vi "SPI Set Frame Size.vi"(8 "Error In":errorcluster, 9 "Frame Size (Bytes)":u8, 10 "SPI Channel (0)":u8, 11 "LINX Device Config":T1) -> (0 "Error Out":errorcluster, 3 "LINX Device Config":T1)   [LabVIEW 2020, in "LMH-LINX.lvlib" / "Device.lvlib"]
doc: "Set the frame size in bytes for the specified SPI Channel."
uses:
  Device.lvlib
  Type Defs/LINX Device Config.ctl
  Type Defs/Interface.ctl
  Type Defs/TCP Config.ctl
  Type Defs/Channels.ctl
  Type Defs/Error Type.ctl
  LMH-LINX.lvlib
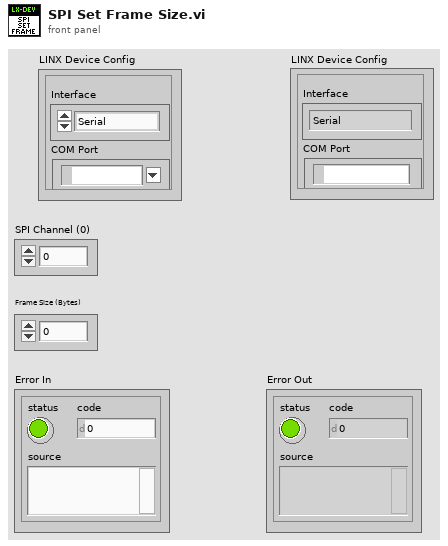
[diagram p1: front panel]
types:
  T1 = typedef "LMH-LINX.lvlib/Device.lvlib/LINX Device Config.ctl" = cluster{"Interface":T2, "COM Port":refnum<visa-resource-name>, "TCP Configuration":T3, "Device Family":u8, "Device ID":u8, "Device Name":string, "TCP Ref":refnum<k5>, "Channels":T4}
  T2 = typedef "LMH-LINX.lvlib/Interface.ctl" = enum16{"Serial", "TCP"}
  T3 = typedef "LMH-LINX.lvlib/Device.lvlib/TCP Config.ctl" = cluster{"IP Address":string, "Port":u16}
  T4 = typedef "LMH-LINX.lvlib/Channels.ctl" = cluster{"DI":u8[], "DO":u8[], "AI":u8[], "AO":u8[], "PWM":u8[], "QE":u8[], "UART":u8[], "I2C 2":u8[], "SPI":u8[], "CAN":u8[], "Servo":u8[], "AI Ref (V)":dbl, "AI Resolution (Bits)":u8, "AO Ref (V)":dbl, "AO Resolution (Bits)":u8}
  T5 = typedef "LMH-LINX.lvlib/Error Type.ctl" = enum16{"Unknown", "Timeout", "Corrupt Return Packet", "Unable To Connect", "Command Not Supported", "Channel DNE", "Invalid COM Config", "Firmware Version Mismatch", "myRIO Support", "CMD Specific Error", "Local IO Not Supported"}
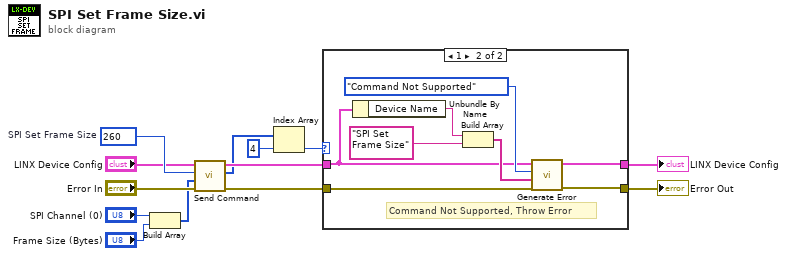
[diagram p0: block diagram]
diagram:
  w12 = u16 260  # SPI Set Frame Size
  n1 = Build Array("SPI Channel (0)", "Frame Size (Bytes)") -> (w5:u8[])
  n2 = call "Send Command.vi"("Error In"="Error In", "ARGS"=w5, "CMD"=w12, "LINX Device Config"="LINX Device Config") -> ("Error Out"=w7:errorcluster, "Response"=w4:u8[], "LINX Device Config"=w9:T1)  [unwired: 4 in, 1 out]
  n3 = Index Array(array=w4, index=4) -> (element=w2:u8)
  n4 = case shown="1" w2 {
    tunnel: [w15 w21] -> w10
    tunnel: w9 -> [w15 w17]
    tunnel: [w14 w22] -> w8
    tunnel: w7 -> [w14 w23]
    frame 0, Default {
      # "Status OK, Process Data"
    }
    frame 1 {
      # "Command Not Supported, Throw Error"
      n5 = Unbundle By Name(w17) -> ("Device Name"=w16:string)
      n6 = Build Array(w16, "SPI Set Frame Size") -> (w18:string[])
      n7 = call "Generate Error.vi"("Error In"=w23, "Arguments"=w18, "Error Type"=Error_Type."Command Not Supported", "LINX Device Config"=w17) -> ("Error Out"=w22:errorcluster, "Dup LINX Device Config"=w21:T1)  [unwired: 6 in]
    }
  }
  "Error Out" <- w8
  "LINX Device Config" <- w10
